vi "SingleFloat (Scalar) to String.vi"(7 "Use System Default Notation (F)":bool, 11 "Value (Single)":sgl format="%#_7g") -> (3 "Value (String)":string)   [LabVIEW 2013, in "OpenScalar.lvlib"]
uses:
  OpenScalar.lvlib
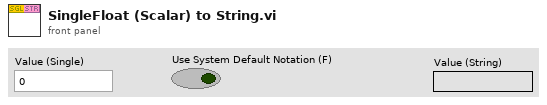
[diagram p1: front panel]
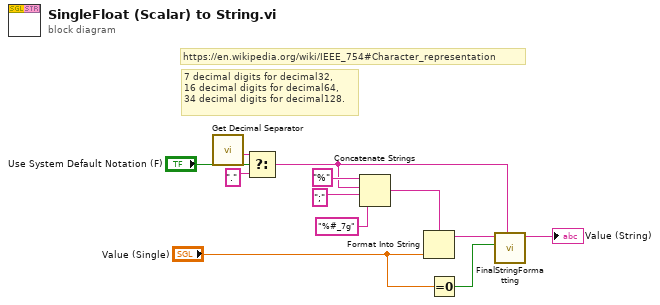
[diagram p0: block diagram]
diagram:
  # "7 decimal digits for decimal32,\n16 decimal digits for decimal64,\n34 decimal digits for decimal128."
  # "https://en.wikipedia.org/wiki/IEEE_754#Character_representation"
  n1 = call "Get Decimal Separator.vi"() -> ("System Decimal separator"=w9:string)  [unwired: 11 in]
  n2 = Select(t=w9, s="Use System Default Notation (F)", f="." ("format string")) -> (s? t:f=w5:string)
  n3 = Concatenate Strings("%" ("format string"), w5, ";" ("regular expression"), "%#_7g" ("format string")) -> (w6:string)
  n4 = Format Into String(format string=w6, "Value (Single)") -> (resulting string=w4:string)  [unwired: 2 in, 1 out]
  n5 = Equal To 0?(x="Value (Single)") -> (x = 0?=w1:bool)
  n6 = call "FinalStringFormatting.vi"("Decimal Notation (.)"=w5, "Equals Zero?"=w1, "String in"=w4) -> ("String out"=→"Value (String)":string)  [unwired: 8 in]
